vi "ASrreglo0disp.vi"(4 "datos":dbl[][](array[numeric])) -> (2 "output array":dbl[][](array[numeric]))   [LabVIEW 2016]
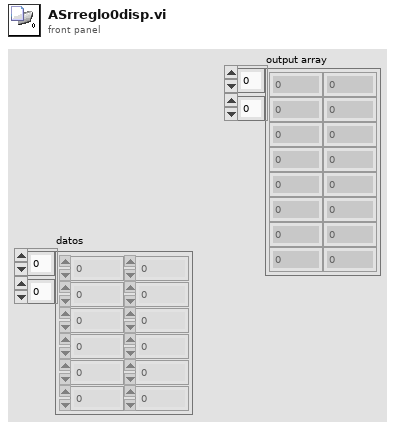
[diagram p1: front panel]
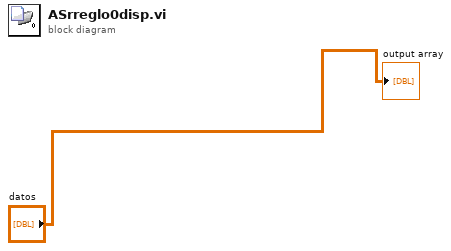
[diagram p0: block diagram]
diagram:
  "output array" <- "datos"
